vi "Identity Value.vi"(3 "Redlines Identity in":refnum<class "Redlines Identity.lvclass">) -> (1 "Value":string)   [LabVIEW 2020, in "VolatusData.lvlib" / "Redlines Identity.lvclass"]
uses:
  Redlines Identity.lvclass
  Redlines Identity.lvclass/Redlines Identity.ctl
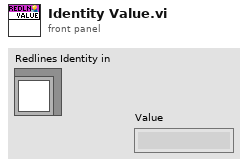
[diagram p1: front panel]
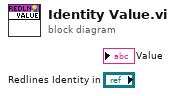
[diagram p0: block diagram]
diagram:
